vi "Info button.vi"(7 "TipPanelHandle":refnum<class "TipPanelHandle.lvclass">, 11 "Info":bool) -> ()   [LabVIEW 2021, in "RocketPlot.lvlib"]
uses:
  RocketPlot.lvlib
  <userlib>/bjustice/TipStripOOPanel/Classes/TipPanelHandle/TipPanelHandle.lvclass
  Classes/TipTablePanel/TipTablePanel.lvclass
  C:/Program Files/National Instruments/LabVIEW 2021/user.lib/bjustice/TipStripOOPanel/Classes/TipPanel/TipPanel.lvclass
  Classes/RocketPlotShortcuts/RocketPlotShortcuts.lvclass
  <userlib>/bjustice/TipStripOOPanel/Classes/TipPanelHandle/CMD - show panel.vi
  C:/Program Files/National Instruments/LabVIEW 2021/vi.lib/IlluminatedG/IG OOPanel/OOPanel/Panel/Panel.lvclass
  C:/Users/bjustice/Documents/GitHub/BluePlot/Source/Classes/TipTablePanel/TipTablePanel.lvclass
  C:/Users/bjustice/Documents/GitHub/BluePlot/Source/Classes/RocketPlotShortcuts/RocketPlotShortcuts.lvclass
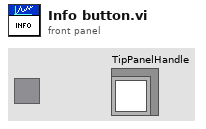
[diagram p1: front panel]
types:
  T1 = typedef "RocketPlot.lvlib/TipTablePanel.lvclass/cell cache.ctl" = cluster{"text":string, "Color":u32, "Justification":enum16{"Left", "Center", "Right"}}
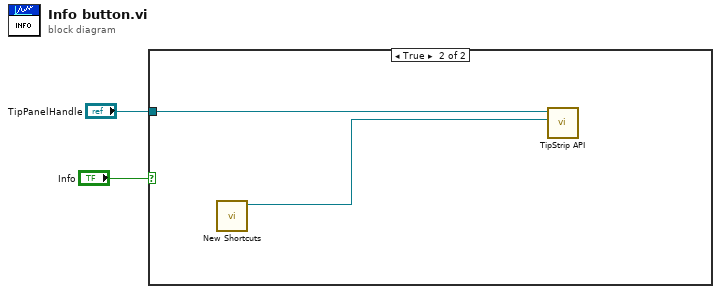
[diagram p0: block diagram]
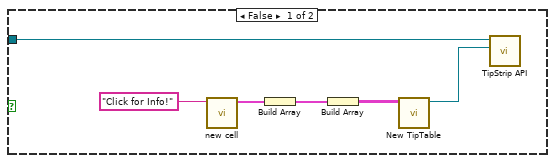
[diagram p2: hidden frame]
diagram:
  n1 = case shown="True" "Info" {
    tunnel: "TipPanelHandle" -> [w4 w10]
    frame False {
      n2 = call "new cell.vi"("String"="Click for Info!") -> ("cell"=w6:T1)  [unwired: 10 in]
      n3 = Build Array(w6) -> (w8:T1[])
      n4 = Build Array(w8) -> (w5:T1[][])
      n5 = call "New TipTable.vi"("show.cells"=w5) -> ("TipTablePanel out"=w3:refnum<class "TipTablePanel.lvclass">)  [unwired: 9 in, 1 out]
      n6 = call-poly <userlib>:"TipStrip API.vi"("TipPanel"=w3, "TipPanelHandle"=w4) -> ()  [unwired: 8 in, 2 out]
    }
    frame True {
      n7 = call "New Shortcuts.vi"() -> ("StokePlotShortcuts out"=w9:refnum<class "RocketPlotShortcuts.lvclass">)  [unwired: 10 in, 1 out]
      n8 = call-poly <userlib>:"TipStrip API.vi"("TipPanel"=w9, "TipPanelHandle"=w10) -> ()  [unwired: 8 in, 2 out]
    }
  }
